vi "P8_modulo_fase.vi"() -> ()   [LabVIEW 2020]
uses:
  <vilib>/vision/NI_Vision_Development_Module.lvlib
panel:
  in  "File Path 2":path=path "D:/usuarios/aif/Docencia/TDS grado/TDS_Tecnologias/P8 DFT2D/cameraman.tif"
  in  "File Path":path=path "D:/usuarios/aif/Docencia/TDS grado/TDS_Tecnologias/P8 DFT2D/lenna.tif"
  out "imagen 2 bis 5":T1(plugin-control)
  out "fft 2":T1(plugin-control)
  out "imagen 1 bis":T1(plugin-control)
  out "fft 1":T1(plugin-control)
  out "Imagen 2":T1(plugin-control)
  out "Imagen 1":T1(plugin-control)
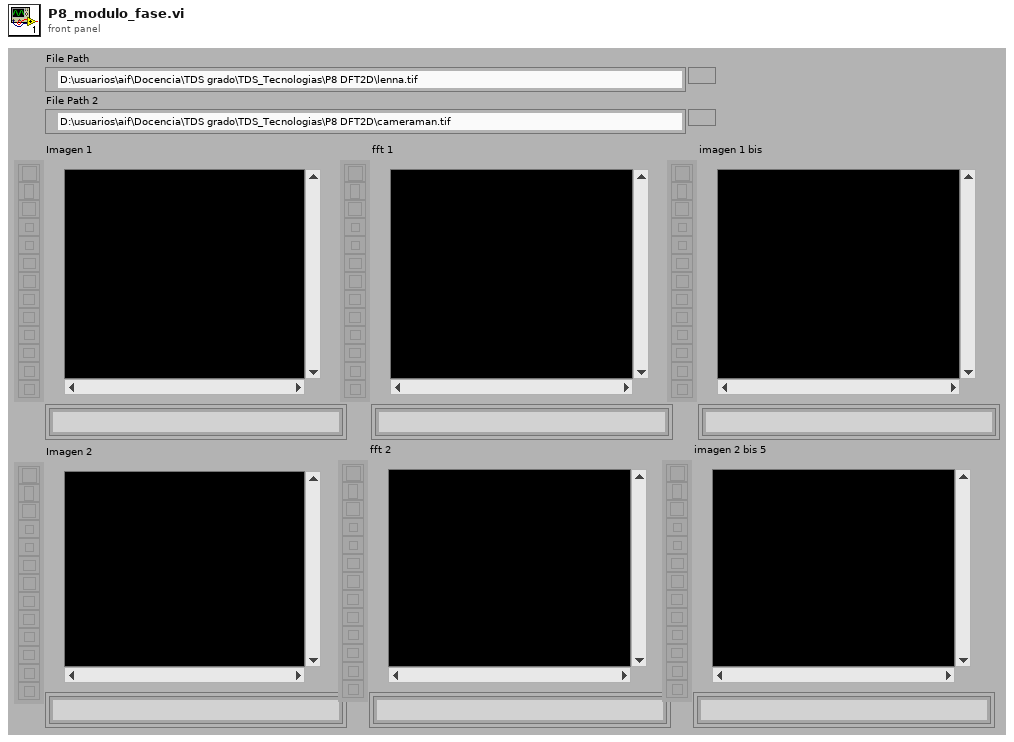
[diagram p1: front panel]
types:
  T1 = typedef "IMAQ Image.ctl" = refnum<image>
  T2 = typedef "Image Type" = u32
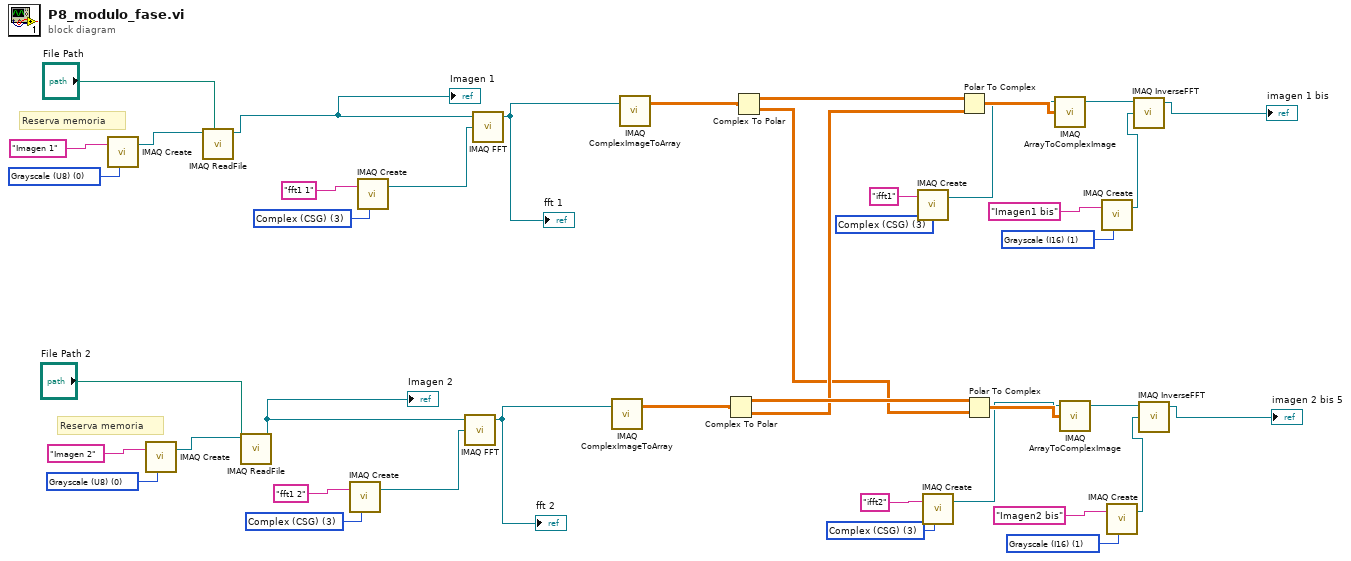
[diagram p0: block diagram]
diagram:
  w6 = T2 1 items=["Grayscale (U8)", "Grayscale (I16)", "Grayscale (SGL)", "Complex (CSG)", "RGB (U32)", "HSL (U32)", "RGB (U64)", "Grayscale (U16)"] ("Image Type")
  w9 = T2 3 items=["Grayscale (U8)", "Grayscale (I16)", "Grayscale (SGL)", "Complex (CSG)", "RGB (U32)", "HSL (U32)", "RGB (U64)", "Grayscale (U16)"] ("Image Type")
  w17 = T2 3 items=["Grayscale (U8)", "Grayscale (I16)", "Grayscale (SGL)", "Complex (CSG)", "RGB (U32)", "HSL (U32)", "RGB (U64)", "Grayscale (U16)"] ("Image Type")
  w21 = T2 1 items=["Grayscale (U8)", "Grayscale (I16)", "Grayscale (SGL)", "Complex (CSG)", "RGB (U32)", "HSL (U32)", "RGB (U64)", "Grayscale (U16)"] ("Image Type")
  w24 = T2 3 items=["Grayscale (U8)", "Grayscale (I16)", "Grayscale (SGL)", "Complex (CSG)", "RGB (U32)", "HSL (U32)", "RGB (U64)", "Grayscale (U16)"] ("Image Type")
  w33 = T2 3 items=["Grayscale (U8)", "Grayscale (I16)", "Grayscale (SGL)", "Complex (CSG)", "RGB (U32)", "HSL (U32)", "RGB (U64)", "Grayscale (U16)"] ("Image Type")
  w38 = T2 0 items=["Grayscale (U8)", "Grayscale (I16)", "Grayscale (SGL)", "Complex (CSG)", "RGB (U32)", "HSL (U32)", "RGB (U64)", "Grayscale (U16)"] ("Image Type")
  w39 = T2 0 items=["Grayscale (U8)", "Grayscale (I16)", "Grayscale (SGL)", "Complex (CSG)", "RGB (U32)", "HSL (U32)", "RGB (U64)", "Grayscale (U16)"] ("Image Type")
  # "Reserva memoria"
  # "Reserva memoria"
  n1 = call "IMAQ Create"("Image Name"="Imagen 1", "Image Type"=w39) -> ("New Image"=w40:T1)  [unwired: 2 in, 2 out]
  n2 = call "IMAQ Create"("Image Name"="Imagen 2", "Image Type"=w38) -> ("New Image"=w37:T1)  [unwired: 2 in, 2 out]
  n3 = call "IMAQ ReadFile"("File Path"="File Path", "Image"=w40) -> ("Image Out"=w32:T1)  [unwired: 3 in, 6 out]
  "Imagen 1" <- w32
  n4 = call "IMAQ ReadFile"("File Path"="File Path 2", "Image"=w37) -> ("Image Out"=w3:T1)  [unwired: 3 in, 6 out]
  "Imagen 2" <- w3
  n5 = call "IMAQ Create"("Image Name"="fft1 2", "Image Type"=w17) -> ("New Image"=w16:T1)  [unwired: 2 in, 2 out]
  n6 = call "IMAQ Create"("Image Name"="fft1 1", "Image Type"=w33) -> ("New Image"=w31:T1)  [unwired: 2 in, 2 out]
  n7 = call "IMAQ FFT"("Image Dst"=w16, "Image Src"=w3) -> ("Image Dst Out"=w15:T1)  [unwired: 1 in, 2 out]
  "fft 2" <- w15
  n8 = call "IMAQ FFT"("Image Dst"=w31, "Image Src"=w32) -> ("Image Dst Out"=w30:T1)  [unwired: 1 in, 2 out]
  "fft 1" <- w30
  n9 = call "IMAQ ComplexImageToArray"("Image"=w15) -> ("Image Pixels (Complex)"=w14:csg[][])  [unwired: 2 in, 3 out]
  n10 = call "IMAQ ComplexImageToArray"("Image"=w30) -> ("Image Pixels (Complex)"=w29:csg[][])  [unwired: 2 in, 3 out]
  n11 = Complex To Polar(r * e^(i*theta)=w14) -> (r=w11:sgl[][], theta=w2:sgl[][])
  n12 = Complex To Polar(r * e^(i*theta)=w29) -> (r=w26:sgl[][], theta=w1:sgl[][])
  n13 = call "IMAQ Create"("Image Name"="ifft1", "Image Type"=w24) -> ("New Image"=w23:T1)  [unwired: 2 in, 2 out]
  n14 = call "IMAQ Create"("Image Name"="ifft2", "Image Type"=w9) -> ("New Image"=w8:T1)  [unwired: 2 in, 2 out]
  n15 = Polar To Complex(1:w2, 2:w26) -> (0:w27:csg[][])
  n16 = Polar To Complex(1:w1, 2:w11) -> (0:w12:csg[][])
  n17 = call "IMAQ ArrayToComplexImage"("Image Pixels (Complex)"=w27, "Image"=w23) -> ("Image Out"=w28:T1)  [unwired: 1 in, 2 out]
  n18 = call "IMAQ ArrayToComplexImage"("Image Pixels (Complex)"=w12, "Image"=w8) -> ("Image Out"=w13:T1)  [unwired: 1 in, 2 out]
  n19 = call "IMAQ Create"("Image Name"="Imagen1 bis", "Image Type"=w21) -> ("New Image"=w20:T1)  [unwired: 2 in, 2 out]
  n20 = call "IMAQ Create"("Image Name"="Imagen2 bis", "Image Type"=w6) -> ("New Image"=w5:T1)  [unwired: 2 in, 2 out]
  n21 = call "IMAQ InverseFFT"("Image Dst"=w20, "Image Src"=w28) -> ("Image Dst Out"=→"imagen 1 bis":T1)  [unwired: 1 in, 2 out]
  n22 = call "IMAQ InverseFFT"("Image Dst"=w5, "Image Src"=w13) -> ("Image Dst Out"=→"imagen 2 bis 5":T1)  [unwired: 1 in, 2 out]
